vi "Sweep_mode.vi"(2 "fast_mode":u16[](array[numeric])) -> (0 "ramp?":bool, 1 "Sweep mode":enum16{"Normal sweep", "Fast sweep"}(ring))   [LabVIEW 2013]
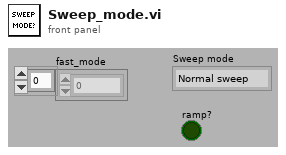
[diagram p1: front panel]
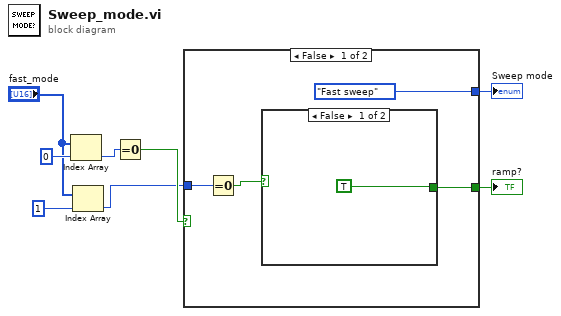
[diagram p0: block diagram]
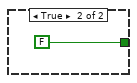
[diagram p2: hidden frame]
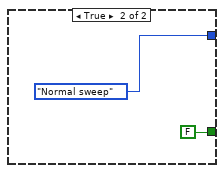
[diagram p3: hidden frame]
diagram:
  n1 = Index Array(array="fast_mode", index=0) -> (element=w7:u16)
  n2 = Index Array(array="fast_mode", index=1) -> (element=w4:u16)
  n3 = Equal To 0?(x=w7) -> (x = 0?=w6:bool)
  n4 = case shown="False" w6 {
    tunnel: w4 -> [w12 _]
    tunnel: [enum16{"Normal sweep", "Fast sweep"}."Fast sweep" enum16{"Normal sweep", "Fast  sweep"}."Normal sweep"] -> w2
    tunnel: [w9 FALSE] -> w1
    frame False {
      n5 = Equal To 0?(x=w12) -> (x = 0?=w11:bool)
      n6 = case shown="False" w11 {
        tunnel: [TRUE ("ramp?") FALSE ("ramp?")] -> w9
        frame False {
        }
        frame True {
        }
      }
    }
    frame True {
    }
  }
  "Sweep mode" <- w2
  "ramp?" <- w1
